vi "add_only_string_on_bd.vi"(8 "error in":errorcluster, 10 "Instrument Command":string, 11 "VI Ref In":refnum<vi>) -> (0 "error out":errorcluster, 3 "VI Ref Out":refnum<vi>)   [LabVIEW 2018]
uses:
  Misc/AddNode/TypeDefinitions/node_types.ctl
  Iternl/CalPos/CmdToStr/TypeDefinitions/main_position_types.ctl
  Iternl/GetNodeTerm/StringProcessingNode/TypeDefinitions/string_node_type.ctl
  Iternl/ConttWire/TypeDefines/connect_with_last_node_types.ctl
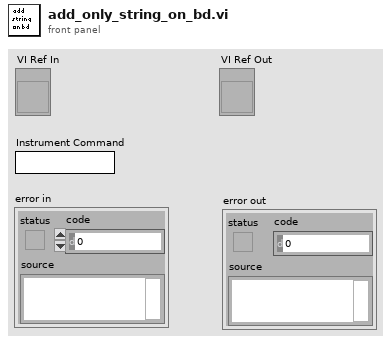
[diagram p1: front panel]
types:
  T1 = typedef "string_node_type.ctl" = enum16{"FormatIntoString", "PickLine", "AppendTrueFalse", "ConcatenateStrings"}
  T2 = typedef "node_types.ctl" = enum16{"FormatIntoString", "PickLine", "AppendTrueFalse", "VISAWrite", "SubVI", "ConcatenateStrings", "VISARead", "ProperyNode", "ScanFromString", "SpreadSheetStringToArray"}
  T3 = typedef "main_position_types.ctl" = enum16{"Node", "FormatNodeForMultipleControls", "BoolConstant", "FormatConstant", "1stSubNodeX"}
  T4 = typedef "connect_with_last_node_types.ctl" = u16
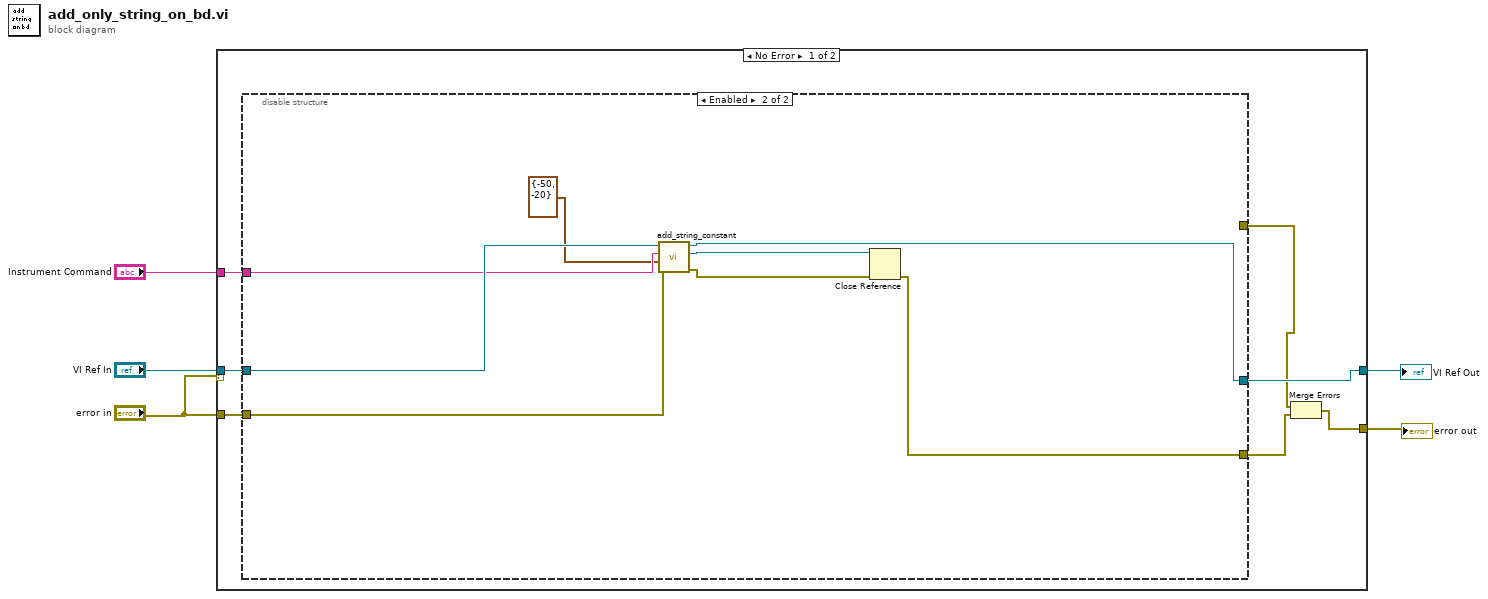
[diagram p0: block diagram]
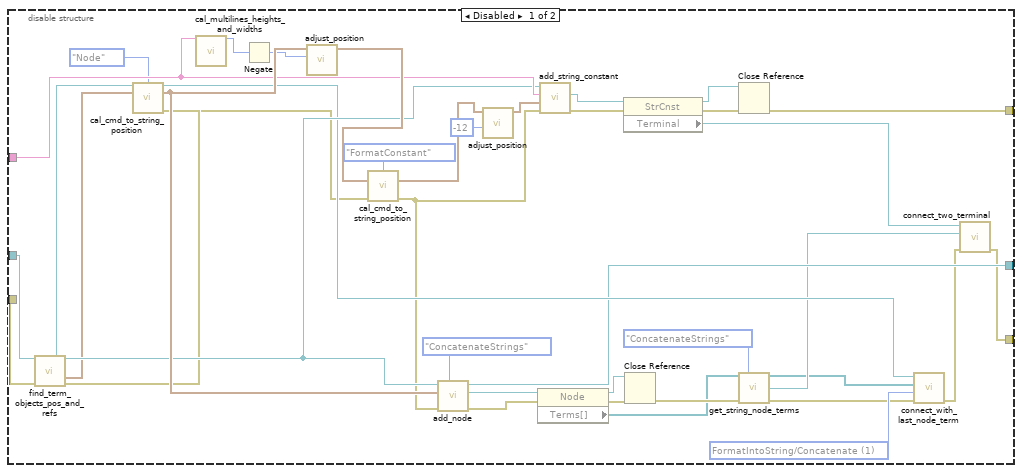
[diagram p2: hidden frame]
diagram:
  n1 = case shown="No Error" "error in" {
    selector: "error in" -> [_ w62]
    tunnel: "Instrument Command" -> [w12 _]
    tunnel: "error in" -> [w11 _]
    tunnel: [w10 w61] -> w4
    tunnel: "VI Ref In" -> [w9 w61]
    tunnel: [w7 w62] -> w2
    frame No Error {
      n2 = disable-structure shown="Enabled" {
        disable-tunnel: w12 -> [w48 w59]
        disable-tunnel: w11 -> [w33 w58]
        disable-tunnel: [w32 w54] -> w10
        disable-tunnel: w9 -> [w31 w60]
        disable-tunnel: [w30 _] -> w8
        disable-tunnel: [w13 w53] -> w6
        frame Disabled {
          w25 = T4 1 items=["AppendTrueFalseString/VisaWrite"=4, "PickLine"=3, "FormatIntoString/Concatenate"=1] ("Terminal Index")
          n3 = call "find_term_objects_pos_and_refs.vi"("VI Ref In"=w31, "error in (no error)"=w33) -> ("Last Function"=w42:refnum<vi>, "VI Ref Out"=w46:refnum<vi>, "Last Function Position"=w40:cluster{"Left":i32, "Top":i32}, "error out"=w39:errorcluster)  [unwired: 10 out]
          n4 = call "cal_cmd_to_string_position.vi"("Last Function Ref In"=w42, "Enum"=main_position_types."Node", "Main Node BD Position"=w40, "error in (no error)"=w39) -> ("Last Function Ref Out"=w43:refnum<vi>, "Main Node Position/Enable Constant Position"=w51:cluster{"Left":u32, "Top":i32}, "error out"=w34:errorcluster)  [unwired: 3 in, 6 out]
          n5 = call "cal_multilines_heights_and_widths.vi"("Ring Command"=w48) -> ("BD Width"=w49:i32)  [unwired: 5 in, 9 out]
          n6 = Negate(x=w49) -> (-x=w50:i32)
          n7 = call "adjust_position.vi"("X Offset"=w50, "Position In"=w51) -> ("Position Out"=w52:cluster{"Left":i32, "Top":i32})  [unwired: 1 in, 8 out]
          n8 = call "cal_cmd_to_string_position.vi"("Enum"=main_position_types."FormatConstant", "Main Node BD Position"=w52, "error in (no error)"=w34) -> ("Main Node Position/Enable Constant Position"=w29:cluster{"Left":u32, "Top":i32}, "error out"=w41:errorcluster)  [unwired: 4 in, 7 out]
          n9 = call "add_node.vi"("Node Type"=node_types."ConcatenateStrings", "error in (no error)"=w41, "BD Position"=w51, "VI Ref In"=w46) -> ("error out"=w14:errorcluster, "Node Refnum"=w21:refnum<vi>, "VI Ref Out"=w32:refnum<vi>)  [unwired: 2 in, 3 out]
          n10 = call "adjust_position.vi"("Y Offset"=-12, "Position In"=w29) -> ("Position Out"=w27:cluster{"Left":i32, "Top":i32})  [unwired: 1 in, 8 out]
          n11 = property class="Node"(reference=w21, error in=w14) -> (reference out=w16:refnum<vi>, error out=w17:errorcluster, "Terms[]"=w15:refnum<vi>[])
          n12 = call "add_string_constant.vi"("error in"=w41, "BD Position"=w27, "StringConstantValue"=w48, "VI Ref In"=w46) -> ("error out"=w35:errorcluster, "StrCnst Refnum"=w36:refnum<vi>)  [unwired: 6 out]
          n13 = property class="StrCnst"(reference=w36, error in=w35) -> (reference out=w37:refnum<vi>, error out=w38:errorcluster, "Terminal"=w47:refnum<vi>)
          n14 = Close Reference(reference=w16, error in (no error)=w17) -> (error out=w18:errorcluster)
          n15 = Close Reference(reference=w37, error in (no error)=w38) -> (error out=w30:errorcluster)
          n16 = call "get_string_node_terms.vi"("Terms[] In"=w15, "Node Type"=string_node_type."ConcatenateStrings", "error in (no error)"=w18) -> ("Terms[]  Out"=w19:refnum<vi>[], "Multiline Term/Enable Term/Concantenate Term"=w24:refnum<vi>, "error out"=w20:errorcluster)  [unwired: 1 in, 9 out]
          n17 = call "connect_with_last_node_term.vi"("error in (no error)"=w20, "Terminal Index"=w25, "Terminals[]"=w19, "Last Function Ref In"=w43) -> ("error out"=w26:errorcluster)  [unwired: 1 in, 6 out]
          n18 = call "connect_two_terminal.vi"("error in"=w26, "Terminal 2"=w24, "Terminal 1"=w47) -> ("error out"=w13:errorcluster)  [unwired: 1 in, 7 out]
        }
        frame Enabled {
          n19 = call "add_string_constant.vi"("error in"=w58, "BD Position"=cluster{"Left":i32, "Top":i32} {"Left"=-50, "Top"=-20}, "StringConstantValue"=w59, "VI Ref In"=w60) -> ("error out"=w56:errorcluster, "StrCnst Refnum"=w55:refnum<vi>, "VI Ref Out"=w54:refnum<vi>)  [unwired: 5 out]
          n20 = Close Reference(reference=w55, error in (no error)=w56) -> (error out=w53:errorcluster)
        }
      }
      n21 = Merge Errors(w8, w6) -> (w7:errorcluster)
    }
    frame Error {
    }
  }
  "error out" <- w2
  "VI Ref Out" <- w4
